vi "SubAxisParameters.vi"() -> (0 "AxisParameters":string[](array[string]))   [LabVIEW 2020]
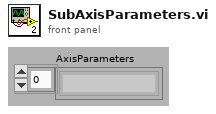
[diagram p1: front panel]
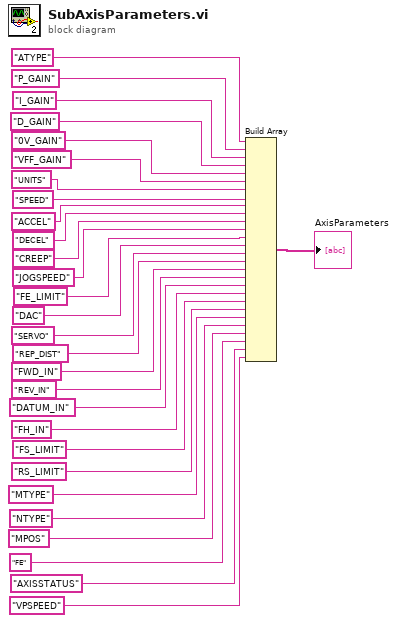
[diagram p0: block diagram]
diagram:
  n1 = Build Array("ATYPE", "P_GAIN", "I_GAIN", "D_GAIN", "0V_GAIN", "VFF_GAIN", "UNITS", "SPEED", "ACCEL", "DECEL", "CREEP", "JOGSPEED", "FE_LIMIT", "DAC", "SERVO", "REP_DIST", "FWD_IN", "REV_IN", "DATUM_IN", "FH_IN", "FS_LIMIT", "RS_LIMIT", "MTYPE", "NTYPE", "MPOS", "FE", "AXISSTATUS", "VPSPEED") -> (→"AxisParameters":string[])
